vi "Galvo Module.vi"(7 "Action":T1(ring)=enum."Calc & Write Scan Pattern", 8 "error in (no error)":errorcluster, 10 "System Parameters":T2={"Optical /HW Parameters"={"Focal Length [mm]"=45.0, "Scan Lens EFL[mm]"=60.0, "Tube Lens EFL[mm]"=180.0, "Galvo V Range (+/-)"=10.0, "Galvo Max Half Angle [Deg]"=19.0, "Max Galvo Range[%]"=0.0}, "Vibratome"={"Z Bottom [mm]"=0.0, "Pre Cut Dwell [s]"=0.0, "Blade Frequency [RPM]"=0, "Slice Speed [mm/s]"=0.0, "Post Cut Dwell [s]"=0.0, "Ramp Time [s]"=0.0, "Start X [mm]"=0.0, "Start Y [mm]"=0.0, "Slice Length [mm]"=0.0, "Slice Axis"=enum."Y Axis", "Controller VISA Ref"="COM4"}, "Table Stages"={"X Stage"={"Position"=0.0, "Is.Enabled?"=FALSE, "Is.Connected?"=FALSE, "Device SN"="45876539", "AccelerationMaximum"=0.0, "VelocityMaximum"=0.0, "Acceleration"=0.0, "Velocity"=0.0, "waitTimeout (ms)"=0, "Model"=enum."None", "Is.Homed?"=FALSE}, "Y Stage"={"Position"=0.0, "Is.Enabled?"=FALSE, "Is.Connected?"=FALSE, "Device SN"="45876539", "AccelerationMaximum"=0.0, "VelocityMaximum"=0.0, "Acceleration"=0.0, "Velocity"=0.0, "waitTimeout (ms)"=0, "Model"=enum."None", "Is.Homed?"=FALSE}, "Z Stage"={"Position"=0.0, "Is.Enabled?"=FALSE, "Is.Connected?"=FALSE, "Device SN"="45876539", "AccelerationMaximum"=0.0, "VelocityMaximum"=0.0, "Acceleration"=0.0, "Velocity"=0.0, "waitTimeout (ms)"=0, "Model"=enum."None", "Is.Homed?"=FALSE}}, "Imaging Parameter"={"Raster Scan Direction"=enum."Uni Directional", "Pixel Dwell Time [Clock Cycles]"=1, "Flyback Time [Clock Cycles]"=10, "XY Center [um]"={"X"=1.0, "Y"=1.0}, "Pixel Step Size [um]"=50.0, "XY Image Resolution"=enum."256 x 256", "Custom"=TRUE, "Custom Size"={"X"=10, "Y"=10}, "Line Averages"=1}} {"Imaging Parameter"."Line Averages" min=1 max=30 step=1; "Imaging Parameter"."Flyback Time [Clock Cycles]" max=10 step=1; "Imaging Parameter"."Pixel Step Size [um]" min=0.0 max=10.0 step=0.01; "Imaging Parameter"."Custom Size"."Y" min=1 max=30 step=1; "Imaging Parameter"."Custom Size"."X" min=1 max=30 step=1; "Imaging Parameter"."XY Center [um]"."Y" min=1.0 max=30.0 step=1.0; "Imaging Parameter"."XY Center [um]"."X" min=1.0 max=30.0 step=1.0; "Imaging Parameter"."Pixel Dwell Time [Clock Cycles]" max=10 step=1}, 11 "Galvo HW Parameters":T6={"Analog Out Channel"="Dev1/ao0", "Min Voltage"=-5.0, "Max Voltage"=5.0, "Pixel Clock Source"="OnboardClock", "Sample Rate"=1000.0, "Line Clock Out Ch"=""}) -> (0 "error out":errorcluster, 1 "task done?":bool)   [LabVIEW 2018]
uses:
  General/Controls/System Parameters.ctl
  Hardware/Table Stage/Controls/Translation Stage Cluster.ctl
  General/Controls/Translation Stage Types.ctl
  General/Controls/Scan Direction.ctl
  <vilib>/DAQmx/write.llb/DAQmx Write (Analog 1D DBL 1Chan NSamp).vi
  <vilib>/DAQmx/write.llb/DAQmx Write (Digital 1D U8 1Chan NSamp).vi
  <vilib>/DAQmx/create/channels.llb/DAQmx Create Channel (AO-Voltage-Basic).vi
  <vilib>/DAQmx/configure/timing.llb/DAQmx Timing (Sample Clock).vi
  <vilib>/DAQmx/miscellaneous.llb/DAQmx Fill In Error Info.vi
  <resource>/objmgr/daqmx.rc
panel:
  # "X"
  # "X"
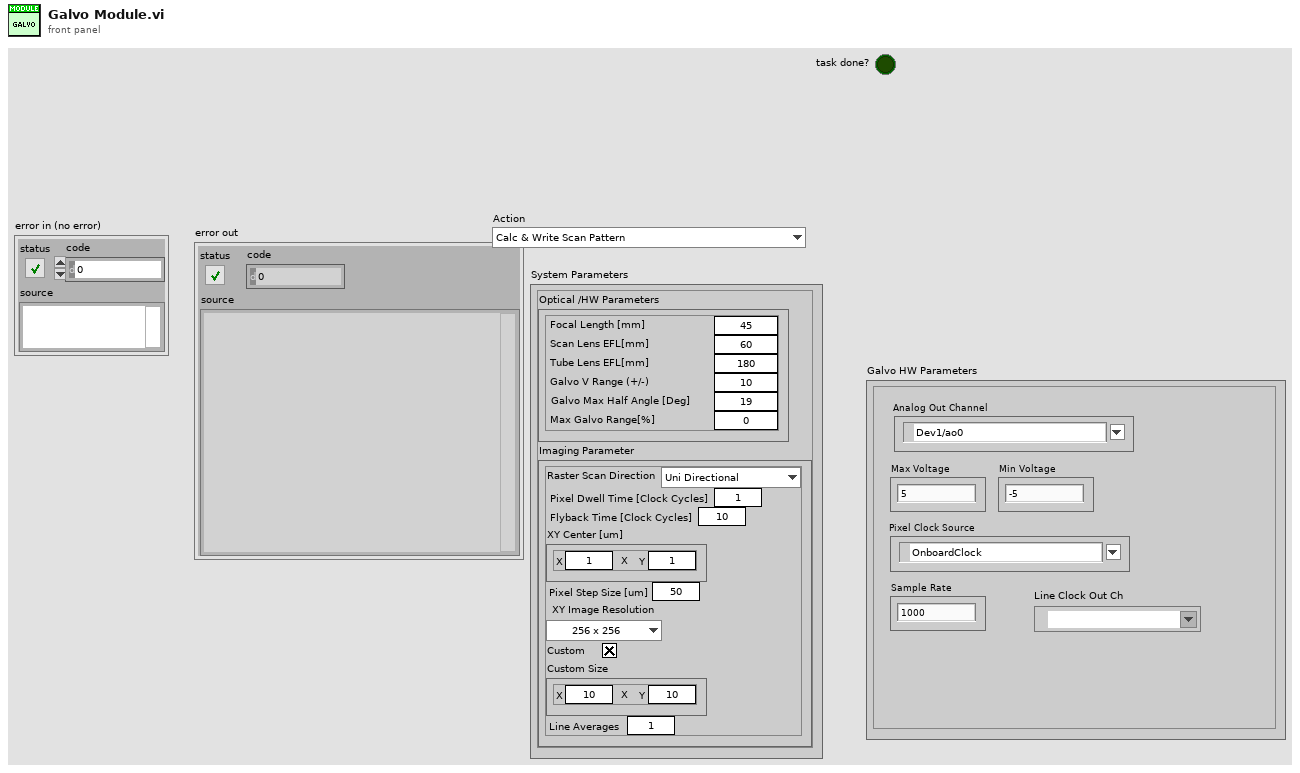
[diagram p1: front panel]
types:
  T1 = enum16{"Init", "Calc & Write Scan Pattern", "Start Galvo Task", "Is Task Done?", "Stop Galvo", "Uninit"}
  T2 = typedef "System Parameters.ctl" = cluster{"Optical /HW Parameters":cluster{"Focal Length [mm]":dbl, "Scan Lens EFL[mm]":dbl, "Tube Lens EFL[mm]":dbl, "Galvo V Range (+/-)":dbl, "Galvo Max Half Angle [Deg]":dbl, "Max Galvo Range[%]":dbl}, "Vibratome":cluster{"Z Bottom [mm]":dbl, "Pre Cut Dwell [s]":dbl, "Blade Frequency [RPM]":u16, "Slice Speed [mm/s]":dbl, "Post Cut Dwell [s]":dbl, "Ramp Time [s]":dbl, "Start X [mm]":dbl, "Start Y [mm]":dbl, "Slice Length [mm]":dbl, "Slice Axis":enum16{"X Axis", "Y Axis", "Z Axis"}, "Controller VISA Ref":refnum<visa-resource-name>}, "Table Stages":cluster{"X Stage":T3, "Y Stage":T3, "Z Stage":T3}, "Imaging Parameter":cluster{"Raster Scan Direction":T5, "Pixel Dwell Time [Clock Cycles]":u16, "Flyback Time [Clock Cycles]":u16, "XY Center [um]":cluster{"X":dbl, "Y":dbl}, "Pixel Step Size [um]":dbl, "XY Image Resolution":enum16{"32 x 32", "64 x 64", "128 x 128", "256 x 256", "512 x 512", "1024 x 1024", "2048 x 2048"}, "Custom":bool, "Custom Size":cluster{"X":u16, "Y":u16}, "Line Averages":u8}}
  T3 = typedef "Translation Stage Cluster.ctl" = cluster{"Position":dbl, "Is.Enabled?":bool, "Is.Connected?":bool, "Device SN":string, "AccelerationMaximum":dbl, "VelocityMaximum":dbl, "Acceleration":dbl, "Velocity":dbl, "waitTimeout (ms)":i32, "Model":T4, "Is.Homed?":bool}
  T4 = typedef "Translation Stage Types.ctl" = enum16{"None", "Thorlabs LTS", "Thorlabs MLJ"}
  T5 = typedef "Scan Direction.ctl" = enum16{"Uni Directional", "Bi Directional", "None"}
  T6 = cluster{"Analog Out Channel":tag, "Min Voltage":dbl, "Max Voltage":dbl, "Pixel Clock Source":tag, "Sample Rate":dbl, "Line Clock Out Ch":tag}
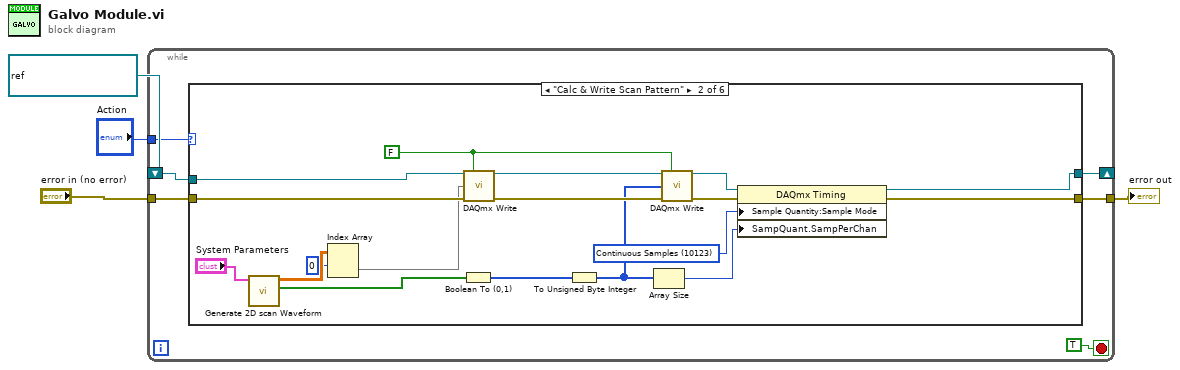
[diagram p0: block diagram]
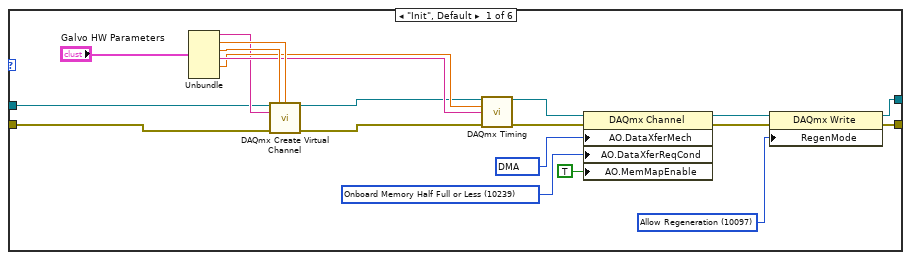
[diagram p2: hidden frame]
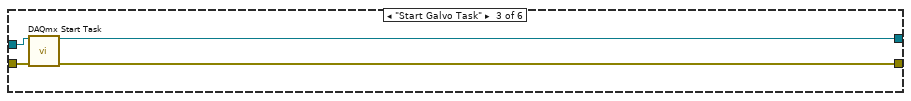
[diagram p3: hidden frame]
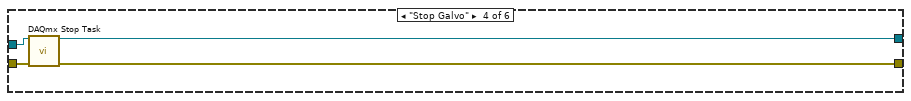
[diagram p4: hidden frame]
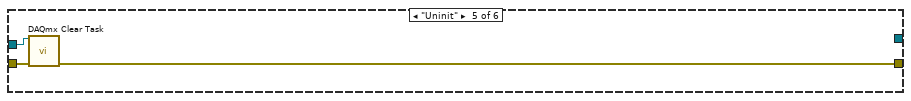
[diagram p5: hidden frame]
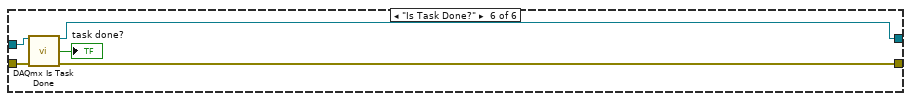
[diagram p6: hidden frame]
diagram:
  n1 = while {
    tunnel: "Action" -> [w10]
    shift-right: [w9] -> _
    shift-left: refnum<k21> "MyVoltageOutTask" ("task out") -> [w8]
    tunnel: [w7] -> w3
    tunnel: "error in (no error)" -> [w6]
    stop <- TRUE stop-if-true
    n2 = case shown="\"Calc & Write Scan Pattern\"" w10 {
      tunnel: [w12 w34 w50 w54 _ w61] -> w9
      tunnel: w8 -> [w11 w46 w51 w55 w58 w63]
      tunnel: [w18 w39 w49 w53 w57 w62] -> w7
      tunnel: w6 -> [w24 w47 w52 w56 w59 w64]
      frame "Init", Default {
        w16 = 10097 items=["Allow Regeneration"=10097, "Do Not Allow Regeneration"=10158] ("RegenMode")
        w20 = 10239 items=["Onboard Memory Empty"=10235, "Onboard Memory Half Full or Less"=10239, "Onboard Memory Less than Full"=10242] ("AO.DataXferReqCond")
        w21 = 10054 items=["DMA"=10054, "Interrupts"=10204, "Programmed I/O"=10264, "USB Bulk"=12590] ("AO.DataXferMech")
        n3 = Unbundle("Galvo HW Parameters") -> ("Analog Out Channel"=w13:tag, "Min Voltage"=w28:dbl, "Max Voltage"=w27:dbl, "Pixel Clock Source"=w26:tag, "Sample Rate"=w25:dbl)  [unwired: 1 out]
        n4 = call-poly <vilib>:"DAQmx Create Virtual Channel.vi"("task in"=w11, "maximum value"=w27, "minimum value"=w28, "physical channels"=w13, "error in"=w24) -> ("task out"=w15:refnum<k21>, "error out"=w14:errorcluster)  [unwired: 9 in]
        n5 = call-poly <vilib>:"DAQmx Timing.vi"("task/channels in"=w15, "rate"=w25, "source"=w26, "error in"=w14) -> ("task out"=w22:refnum<k21>, "error out"=w30:errorcluster)  [unwired: 10 in]
        n6 = property class="DAQmx Channel"(reference=w22, error in=w30, "AO.DataXferMech"=w21, "AO.DataXferReqCond"=w20, "AO.MemMapEnable"=TRUE) -> (reference out=w17:refnum<k21>, error out=w23:errorcluster)
        n7 = property class="DAQmx Write"(reference=w17, error in=w23, "RegenMode"=w16) -> (reference out=w12:refnum<k21>, error out=w18:errorcluster)
      }
      frame "Calc & Write Scan Pattern" {
        w38 = 10123 items=["Finite Samples"=10178, "Continuous Samples"=10123, "Hardware Timed Single Point"=12522] ("SampQuant.SampMode")
        w42 = FALSE ("auto start")
        n8 = call "Generate 2D scan Waveform.vi"("System Parameters [In]"="System Parameters") -> ("Digital Line Acq"=w41:bool[], "Array 3"=w33:dbl[][])  [unwired: 8 in, 1 out]
        n9 = Index Array(array=w33, index (row)=0) -> (element=w31:dbl[])  [unwired: 1 in]
        n10 = Boolean To (0,1)(Boolean=w41) -> (0, 1=w40:i16[])
        n11 = call-poly <vilib>:"DAQmx Write.vi"("task/channels in"=w46, "auto start"=w42, "data"=w31, "error in"=w47) -> ("task out"=w43:refnum<k21>, "error out"=w45:errorcluster)  [unwired: 9 in, 1 out]
        n12 = To Unsigned Byte Integer(number=w40) -> (unsigned 8bit integer=w37:u8[])
        n13 = Array Size(array=w37) -> (size(s)=w36:i32)
        n14 = call-poly <vilib>:"DAQmx Write.vi"("task/channels in"=w43, "auto start"=w42, "data"=w37, "error in"=w45) -> ("task out"=w35:refnum<k21>, "error out"=w44:errorcluster)  [unwired: 9 in, 1 out]
        n15 = property class="DAQmx Timing"(reference=w35, error in=w44, "Sample Quantity:Sample Mode"=w38, "SampQuant.SampPerChan"=w36) -> (reference out=w34:refnum<k21>, error out=w39:errorcluster)
      }
      frame "Start Galvo Task" {
        n16 = call <vilib>:"DAQmx Start Task.vi"("task/channels in"=w51, "error in"=w52) -> ("task out"=w50:refnum<k21>, "error out"=w49:errorcluster)  [unwired: 12 in]
      }
      frame "Stop Galvo" {
        n17 = call <vilib>:"DAQmx Stop Task.vi"("task/channels in"=w55, "error in"=w56) -> ("task out"=w54:refnum<k21>, "error out"=w53:errorcluster)  [unwired: 12 in]
      }
      frame "Uninit" {
        n18 = call <vilib>:"DAQmx Clear Task.vi"("task in"=w58, "error in"=w59) -> ("error out"=w57:errorcluster)  [unwired: 13 in]
      }
      frame "Is Task Done?" {
        n19 = call <vilib>:"DAQmx Is Task Done.vi"("task/channels in"=w63, "error in"=w64) -> ("task out"=w61:refnum<k21>, "task done?"=→"task done?":bool, "error out"=w62:errorcluster)  [unwired: 11 in]
      }
    }
  }
  "error out" <- w3
